vi "ATP_Analysis.vi"(11 "file path (dialog if empty)":path=path "C:/Users/user/Desktop/Andor/ATP") -> (3 "ATP":i32=4060)   [LabVIEW 2020]
uses:
  <vilib>/Utility/file.llb/Write Delimited Spreadsheet (I64).vi
panel:
  in  "Save File":bool
  in  "file path (dialog if empty) 2":path=path "C:/Users/user/Desktop/CO2_Laptop/Data/ATP0201.xls"
  in  "format (%.3f) 2":string="%.5f"
  in  "File Number":i32=1
  in  "Tab Control":enum32{"Page 1", "Page 2"}(tab)=enum."Page 2"
  in  "start of read offset (chars.:0)":i32
  in  "max characters/row  (no limit:0)":i32
  out "mark after read (chars.)":i32=262063
  in  "number of rows (all:-1)":i32=-1
  out "all rows":string[][](array[string])
  in  "format (%.3f)":string="%.3f"
  in  "transpose (no:F)":bool
  in  "type (empty)":string[][](array[string])
  in  "delimiter (Tab)":string=","
  out "EOF?":bool
  out "size(s)":i32[](array[numeric])=[1024, 52]
  in  "index":i32=415
  in  "length":i32=800
  in  "index 2":i32=1
  in  "length 2":i32=43
  out "number":i32[][](array[numeric])
  out "Array":i32[](array[numeric])=[0, 60, 180, 69, 83, 75, 263, 214, 846, 2106, 3665, 4906, 4862, 4375, 4334, 4274, 4141, 4372, 3863, 4034, 4015, 3999, 4378, 4336, 3707, 3655, 4230, 3580, 3973, 3740, 20900, 3771, 3714, 3814, 3720]
  in  "Numeric":i32=35
  out "sorted array2":i32[](array[numeric])=[3863, 3999, 4015, 4034, 4141, 4274, 4334, 4372, 4375, 4378]
  out "sorted array 1":i32[](array[numeric])=[0, 60, 69, 75, 83, 180, 214, 263, 846, 2106, 3665, 4906]
  out "?":cluster{i32[], i32[]}(graph)={[0, 1, 2, 3, 4, 5, 6, 7, 8, 9, 10, 11, 12, 13, 14, 15, 16, 17, 18, 19, 20, 21, 22, 23, 24, 25, 26, 27, 28, 29, 30, 31, 32, 33, 34], [0, 60, 180, 69, 83, 75, 263, 214, 846, 2106, 3665, 4906, 4862, 4375, 4334, 4274, 4141, 4372, 3863, 4034, 4015, 3999, 4378, 4336, 3707, 3655, 4230, 3580, 3973, 3740, 20900, 3771, 3714, 3814, 3720]}
  out "Signal":i32=4274
  out "Background":i32=214
  out "?":cluster{i32[], i32[]}(graph)={[0], [4060]}
  # "ATP with Time"
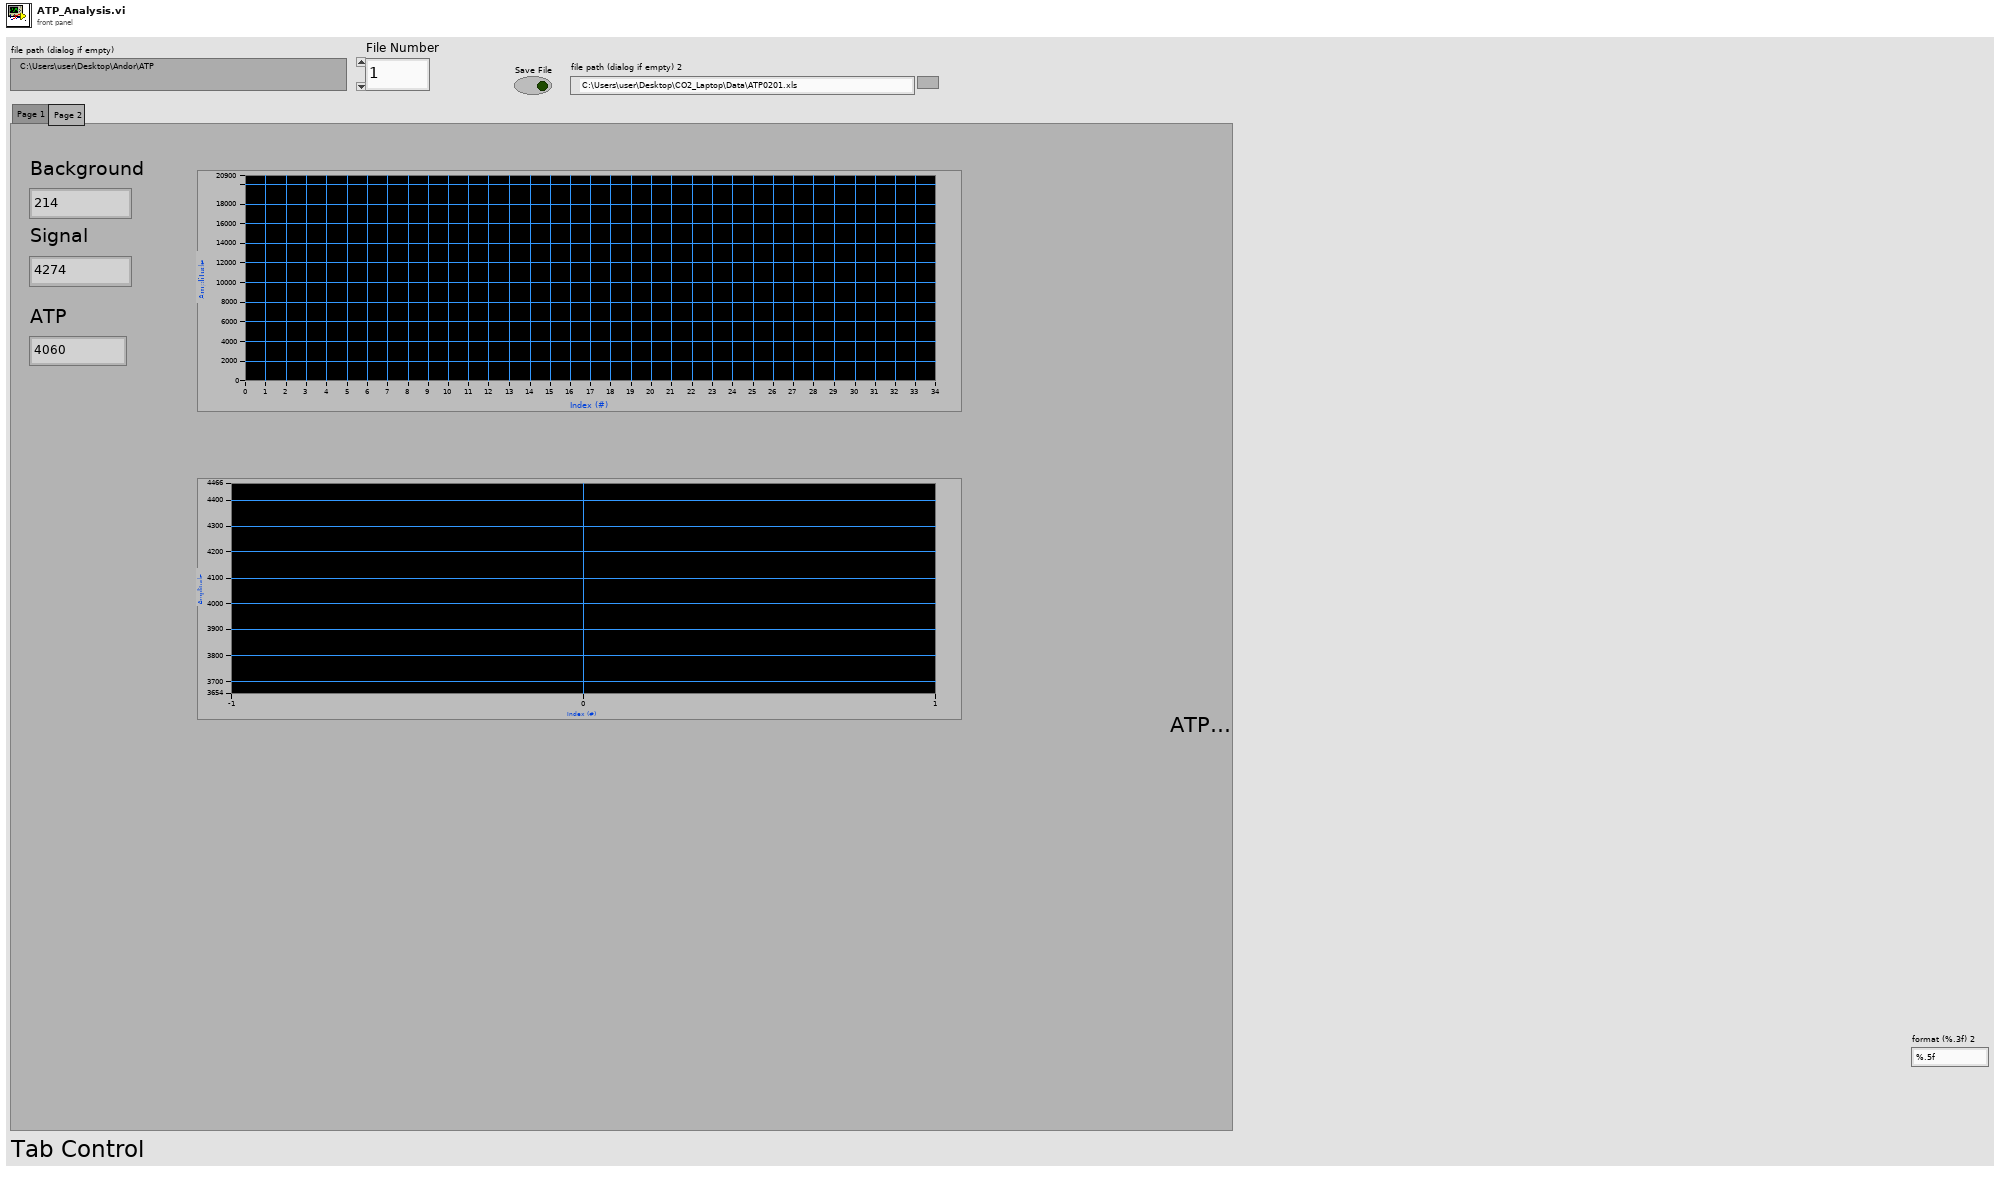
[diagram p1: front panel]
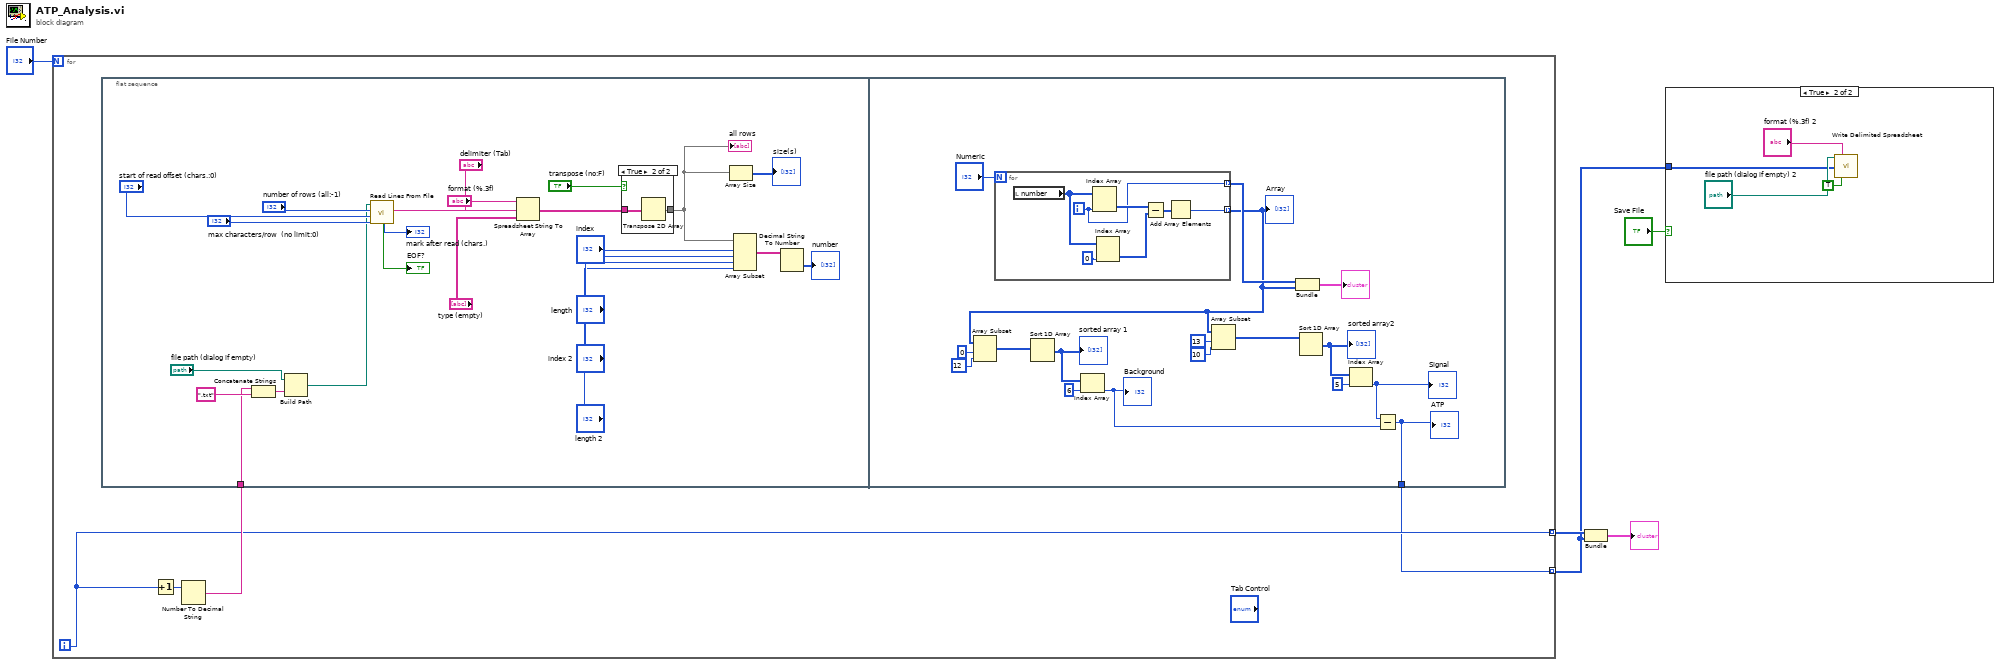
[diagram p0: block diagram]
diagram:
  n1 = for {
    N: "File Number" -> [_]
    tunnel: [w7] -> w3 mode=indexing
    tunnel: [w6] -> w1 mode=indexing
    i -> [w7]
    n2 = flat-sequence {
      tunnel: w8 -> [w10]
      tunnel: [w38] -> w6
      frame #0 {
        n3 = Concatenate Strings(w10, ".txt" ("string")) -> (w14:string)
        n4 = Build Path(base path="file path (dialog if empty)", name or relative path=w14) -> (appended path=w11:path)
        n5 = call <vilib>:"Read Lines From File.vi"("file path (dialog if empty)"=w11, "number of lines (all:-1)"="number of rows (all:-1)", "start of read offset (chars.:0)"="start of read offset (chars.:0)", "[max characters per line]  (no limit:0)"="max characters/row  (no limit:0)") -> ("line string"=w30:string, "mark after read (chars.)"=→"mark after read (chars.)":i32, "EOF?"=→"EOF?":bool)  [unwired: 2 in, 1 out]
        n6 = Spreadsheet String To Array(delimiter (Tab)="delimiter (Tab)", format string="format (%.3f)", spreadsheet string=w30, array type (2D Dbl)="type (empty)") -> (array=w28:string[][])
        n7 = case shown="True" "transpose (no:F)" {
          tunnel: [w34 w36] -> w21
          tunnel: w28 -> [w34 w35]
          frame False {
          }
          frame True {
            n8 = Transpose 2D Array(2D array=w35) -> (transposed array=w36:string[][])
          }
        }
        "all rows" <- w21
        n9 = Array Size(array=w21) -> (size(s)=→"size(s)":i32[])
        n10 = Array Subset(array=w21, index (row)="index", length (row)="length", index (col)="index 2", length (col)="length 2") -> (w16:string[][])
        n11 = Decimal String To Number(string=w16) -> (number=→"number":i32[][])  [unwired: 2 in, 1 out]
      }
      frame #1 {
        n12 = for {
          N: "Numeric" -> [_]
          tunnel: [w60] -> w37 mode=indexing
          tunnel: [w54] -> w52 mode=indexing
          i -> [w54]
          n13 = local read "number"() -> (w58:i32[][])
          n14 = Index Array(array=w58, index (col)=w54) -> (element=w56:i32[])  [unwired: 1 in]
          n15 = Index Array(array=w58, index (col)=0) -> (element=w57:i32[])  [unwired: 1 in]
          n16 = Subtract(x=w56, y=w57) -> (x-y=w55:i32[])
          n17 = Add Array Elements(numeric array=w55) -> (sum=w60:i32)
        }
        "Array" <- w37
        n18 = Array Subset(array=w37, index=0, length=12) -> (w41:i32[])
        n19 = Sort 1D Array(array=w41) -> (sorted array=w43:i32[])
        "sorted array 1" <- w43
        n20 = Index Array(array=w43, index=6) -> (element=w39:i32)
        "Background" <- w39
        n21 = Array Subset(array=w37, index=13, length=10) -> (w48:i32[])
        n22 = Bundle(w52, w37) -> (→"?":cluster{i32[], i32[]})  [unwired: 1 in]
        n23 = Sort 1D Array(array=w48) -> (sorted array=w50:i32[])
        "sorted array2" <- w50
        n24 = Index Array(array=w50, index=5) -> (element=w40:i32)
        "Signal" <- w40
        n25 = Subtract(x=w40, y=w39) -> (x-y=w38:i32)
        "ATP" <- w38
      }
    }
    n26 = Increment(x=w7) -> (x+1=w9:i32)
    n27 = Number To Decimal String(number=w9) -> (decimal integer string=w8:string)  [unwired: 1 in]
  }
  n28 = Bundle(w3, w1) -> (→"?":cluster{i32[], i32[]})  [unwired: 1 in]
  n29 = case shown="True" "Save File" {
    tunnel: w1 -> [_ w62]
    frame False {
    }
    frame True {
      n30 = call-poly <vilib>:"Write Delimited Spreadsheet.vi"("file path (dialog if empty)"="file path (dialog if empty) 2", "format (%d)"="format (%.3f) 2", "1D data"=w62, "transpose? (no:F)"=TRUE) -> ()  [unwired: 10 in, 2 out]
    }
  }
